vi "isEnabled.vi"(8 "error in (no error)":errorcluster, 11 "Tv in":refnum<class "Tv.lvclass">) -> (0 "error out":errorcluster, 2 "on":bool, 3 "Tv out":refnum<class "Tv.lvclass">)   [LabVIEW 2018, in "Tv.lvclass"]
uses:
  Tv.lvclass
  Tv.lvclass/Tv.ctl
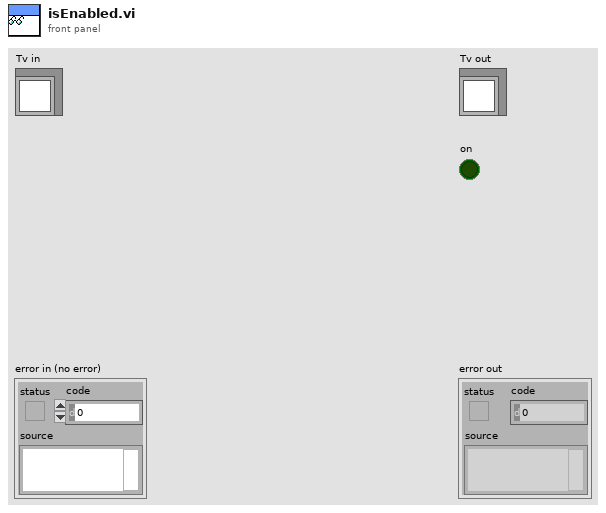
[diagram p1: front panel]
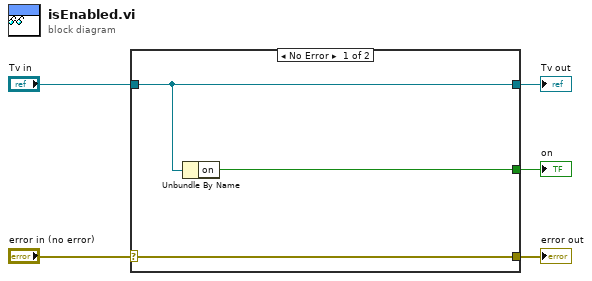
[diagram p0: block diagram]
diagram:
  n1 = case shown="No Error" "error in (no error)" {
    selector: "error in (no error)" -> [w8 w9]
    tunnel: [w8 w9] -> w4
    tunnel: [w7 w10] -> w2
    tunnel: "Tv in" -> [w7 w10]
    tunnel: [w6 _] -> w1
    frame No Error {
      n2 = Unbundle By Name(w7) -> ("on"=w6:bool)
    }
    frame Error {
    }
  }
  "error out" <- w4
  "Tv out" <- w2
  "on" <- w1
